vi "檢測_距離_VI.vi"(8 "error in (no error)":errorcluster, 9 "找圓":cluster{"X":sgl, "Y":sgl}[](array[cluster]), 10 "找邊":cluster{"X":sgl, "Y":sgl}[](array[cluster]), 11 "Image":T1) -> (0 "error out":errorcluster, 1 "Distances":sgl[][](array[numeric]), 2 "min value":sgl, 3 "Image Out":T1)   [LabVIEW 2015]
uses:
  <vilib>/vision/Image Controls.llb/IMAQ Image.ctl
  <vilib>/vision/NI_Vision_Development_Module.lvlib
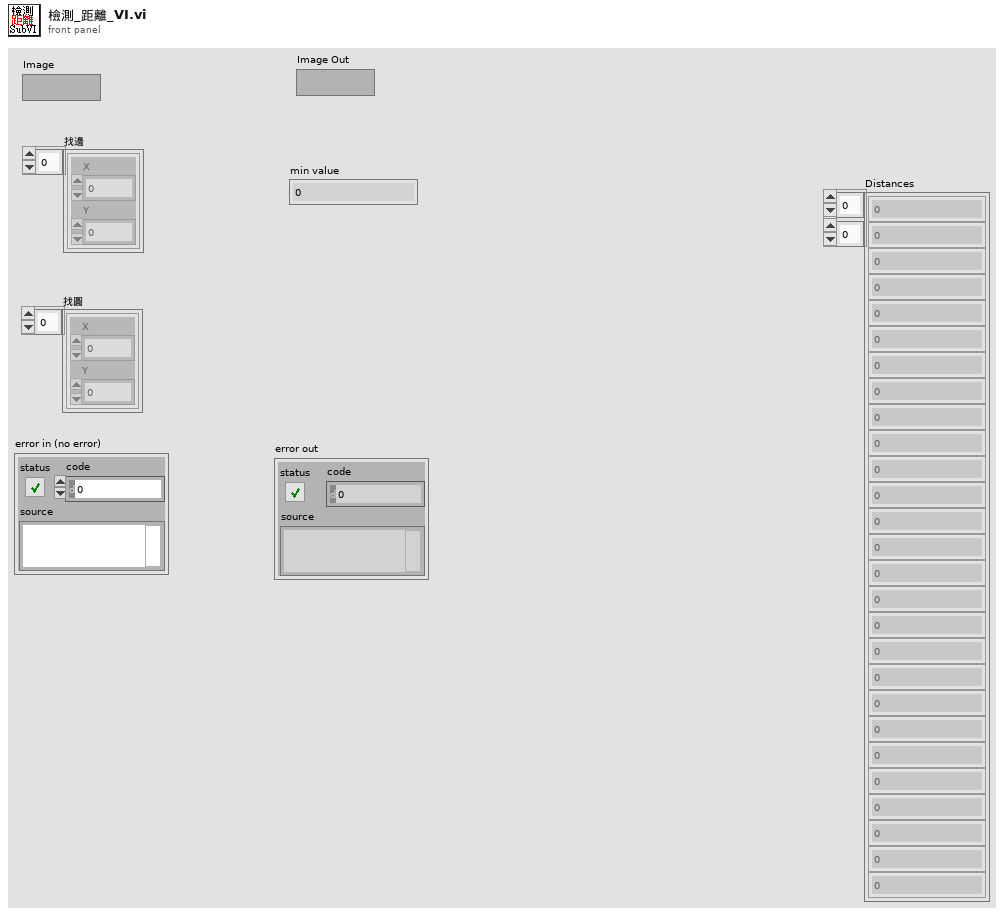
[diagram p1: front panel]
types:
  T1 = typedef "IMAQ Image.ctl" = refnum<image>
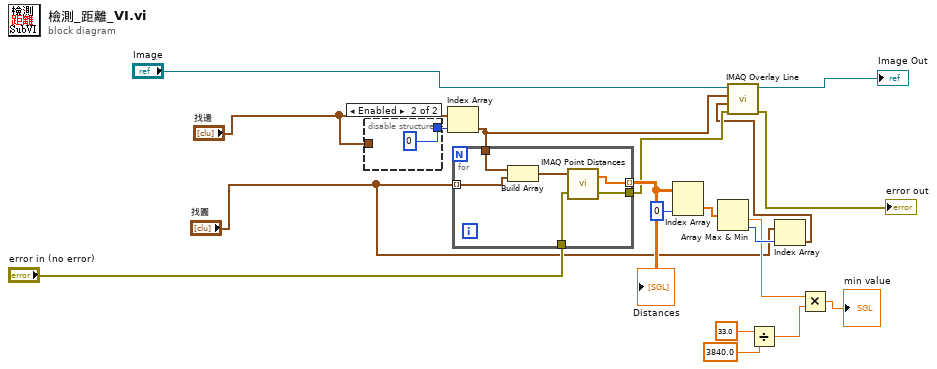
[diagram p0: block diagram]
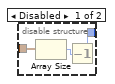
[diagram p2: hidden frame]
diagram:
  n1 = disable-structure shown="Enabled" {
    disable-tunnel: [w21 0] -> w9
    disable-tunnel: "找邊" -> [w20 _]
    frame Disabled {
      n2 = Array Size(array=w20) -> (size(s)=w22:i32)
      n3 = Decrement(x=w22) -> (x-1=w21:i32)
    }
    frame Enabled {
    }
  }
  n4 = Index Array(array="找邊", index=w9) -> (element=w19:cluster{"X":sgl, "Y":sgl})
  n5 = for {
    tunnel: "找圓" -> [w28] mode=indexing
    tunnel: w19 -> [w29]
    tunnel: [w26] -> w16 mode=indexing
    tunnel: "error in (no error)" -> [w25]
    tunnel: [w24] -> w4
    n6 = Build Array(w29, w28) -> (w27:cluster{"X":sgl, "Y":sgl}[])
    n7 = call "IMAQ Point Distances"("Points"=w27, "error in (no error)"=w25) -> ("Distances"=w26:sgl[], "error out"=w24:errorcluster)  [unwired: 3 in]
  }
  "Distances" <- w16
  n8 = Index Array(array=w16, index (col)=0 ("disabled index (col)")) -> (element=w18:sgl[])  [unwired: 1 in]
  n9 = Array Max & Min(array=w18) -> (min value=w14:sgl, min index (indices)=w17:i32)  [unwired: 2 out]
  n10 = Divide(x=33.0, y=3840.0) -> (x/y=w13:dbl)
  n11 = Index Array(array="找圓", index=w17) -> (element=w1:cluster{"X":sgl, "Y":sgl})
  n12 = call "IMAQ Overlay Line"("error in (no error)"=w4, "End Point"=w1, "Start Point"=w19, "Image"="Image") -> ("error out"=→"error out":errorcluster, "Image Out"=→"Image Out":T1)  [unwired: 6 in]
  n13 = Multiply(x=w14, y=w13) -> (x*y=→"min value":dbl)
